vi "main-fan-switch.vi"(7 "LabVIEW Web Service Request":refnum<class "Web Request.lvclass">, 11 "state":bool) -> ()   [LabVIEW 2023]
uses:
  <vilib>/wsapi/Web Request.lvclass
  Actuators.vi
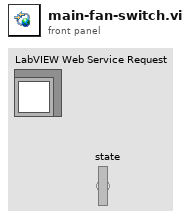
[diagram p1: front panel]
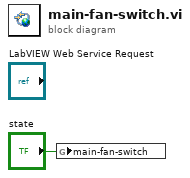
[diagram p0: block diagram]
diagram:
  n1 = global write "Actuators.vi" "main-fan-switch"("state") -> ()
